vi "Populate Result.vi"(8 "error in (no error)":errorcluster, 11 "String Compare in":refnum<class "String Compare.lvclass">) -> (0 "error out":errorcluster, 3 "String Compare out":refnum<class "String Compare.lvclass">)   [LabVIEW 2015, in "String Compare.lvclass"]
doc: "This VI Gathers the information from the step and builds a result with it."
uses:
  String Compare.lvclass
  classes/Result/Result.lvclass
  String Compare.lvclass/String Compare.ctl
  classes/Step/Execution/Step.lvclass
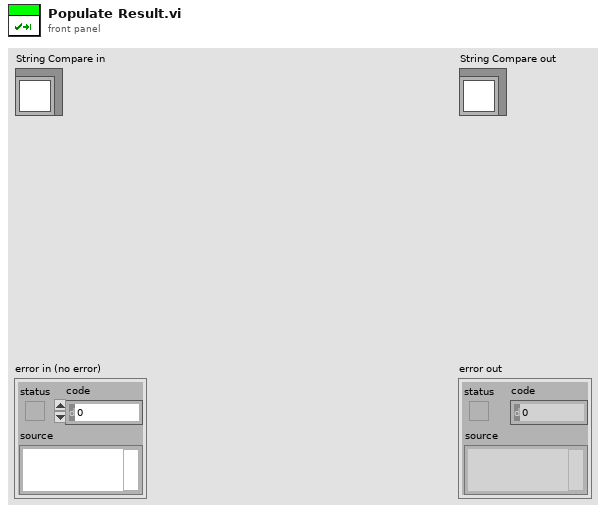
[diagram p1: front panel]
types:
  T1 = typedef "String Compare Config.lvclass/Mode.ctl" = enum16{"Compare Strings", "Match Regex"}
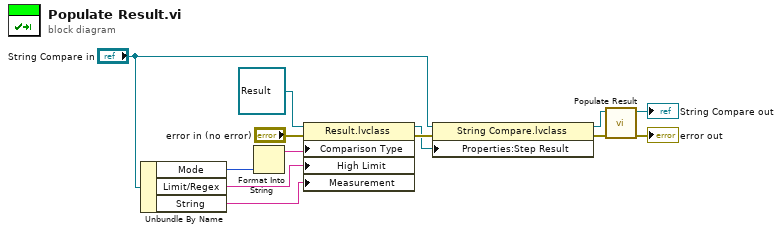
[diagram p0: block diagram]
diagram:
  n1 = Unbundle By Name("String Compare in") -> ("Mode"=w4:T1, "Limit/Regex"=w3:string, "String"=w2:string)
  n2 = Format Into String(w4) -> (resulting string=w10:string)  [unwired: 3 in, 1 out]
  n3 = property class="Result.lvclass"(reference=refnum<class "Result.lvclass"> refnum ("Result.lvclass"), error in="error in (no error)", "Comparison Type"=w10, "High Limit"=w3, "Measurement"=w2) -> (reference out=w7:refnum<class "Result.lvclass">, error out=w9:errorcluster)
  n4 = property class="String Compare.lvclass"(reference="String Compare in", error in=w9, "Properties:Step Result"=w7) -> (reference out=w6:refnum<class "String Compare.lvclass">, error out=w8:errorcluster)
  n5 = call-parent "Populate Result.vi"("error in (no error)"=w8, "Step in"=w6) -> ("error out"=→"error out":errorcluster, "Step out"=→"String Compare out":refnum<class "String Compare.lvclass">)  [unwired: 8 in]
